vi "Update Height by Numeric.vi"(4 "Bottom Numeric":sgl, 5 "Logarithm?":bool, 6 "Top Numeric":sgl=100.0, 7 "Active Numeric Ref":refnum<vi>, 8 "error in (no error)":errorcluster, 9 "Numeric Ref Array":refnum<vi>[](array[refnum]), 10 "Color Ref Array":refnum<vi>[](array[refnum]), 11 "Slider Ref Array":refnum<vi>[](array[refnum])) -> (0 "error out":errorcluster)   [LabVIEW 2020, in "3D Plot.lvclass"]
uses:
  3D Plot.lvclass
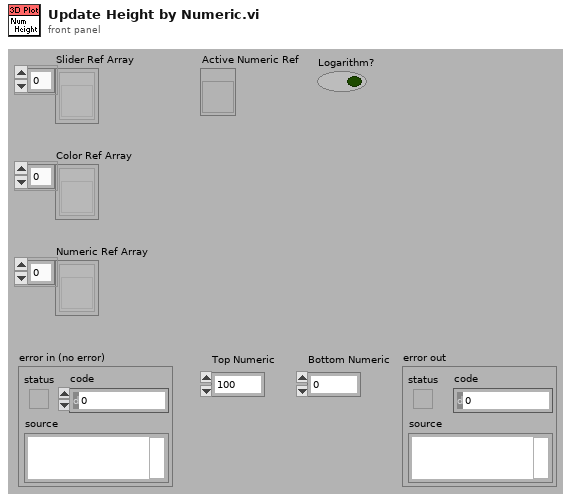
[diagram p1: front panel]
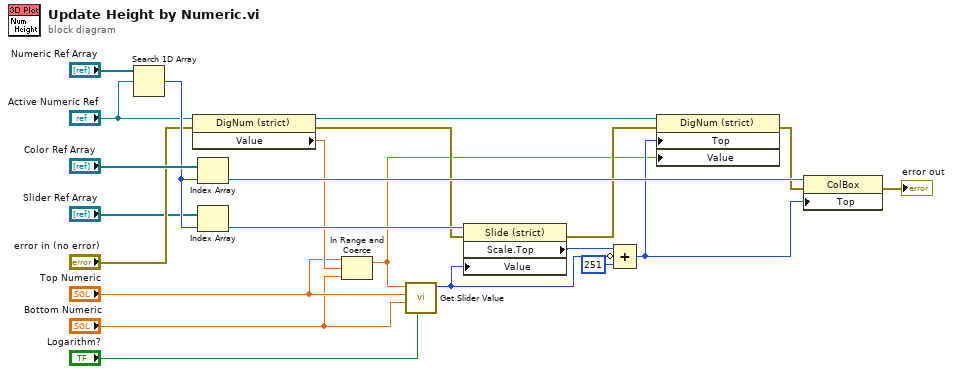
[diagram p0: block diagram]
diagram:
  n1 = Search 1D Array(1D array="Numeric Ref Array", element="Active Numeric Ref") -> (index of element=w21:i32)  [unwired: 1 out]
  n2 = property class="DigNum (strict)"(reference="Active Numeric Ref", error in="error in (no error)") -> (reference out=w10:refnum<vi>, error out=w8:errorcluster, "Value"=w6:sgl)
  n3 = Index Array(array="Color Ref Array", index=w21) -> (element=w20:refnum<vi>)
  n4 = Index Array(array="Slider Ref Array", index=w21) -> (element=w14:refnum<vi>)
  n5 = In Range and Coerce(upper limit="Top Numeric", x=w6, lower limit="Bottom Numeric") -> (coerced(x)=w3:sgl)  [unwired: 1 out]
  n6 = call "Get Slider Value.vi"("Logarithm?"="Logarithm?", "Bottom Numeric"="Bottom Numeric", "Top Numeric"="Top Numeric", "Current Numeric"=w3) -> ("Current Slider"=w5:i32)  [unwired: 7 out]
  n7 = property class="Slide (strict)"(reference=w14, error in=w8, "Value"=w5) -> (error out=w7:errorcluster, "Scale.Top"=w13:i32)  [unwired: 1 out]
  n8 = Compound Arithmetic op=ADD(w13, invert w5, 251 ("value")) -> (w11:i32)
  n9 = property class="DigNum (strict)"(reference=w10, error in=w7, "Top"=w11, "Value"=w3) -> (error out=w9:errorcluster)  [unwired: 1 out]
  n10 = property class="ColBox"(reference=w20, error in=w9, "Top"=w11) -> (error out=→"error out":errorcluster)  [unwired: 1 out]
